vi "FGV Komponentenreferenzen verwalten.vi"(0 "Referenzen":refnum<vi>[](array[refnum]), 7 "Strings []":string[](array[string]), 11 "error in (no error)":errorcluster caption="Fehler (Eingang, kein Fehler)", 13 "Aktion":T1) -> (15 "error out":errorcluster caption="Fehler (Ausgang)")   [LabVIEW 2020, in "Linearisierung v2.lvlib" / "SpanEinstellungen.lvlib"]
uses:
  SpanEinstellungen.lvlib
  Aktion FGV Komponentenreferenz verwalten.ctl
  Gasteiler/HovaCAL_Interface/Kommunikation/Aktion FGV HovaCAL Interface Autolin.ctl
  Gasteiler/HovaCAL_Interface/Kommunikation/Kommunikation.lvlib
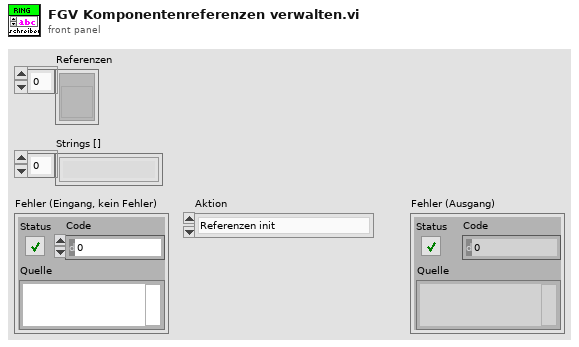
[diagram p1: front panel]
types:
  T1 = typedef "Linearisierung v2.lvlib/SpanEinstellungen.lvlib/Aktion FGV Komponentenreferenz verwalten.ctl" = enum16{"Referenzen init", "lesen", "Referenzen schließen", "Ring beschreiben", "MFC fix Werte setzen"}
  T2 = typedef "Linearisierung v2.lvlib/Gasteiler.lvlib/HovaCAL_Interface.lvlib/Kommunikation.lvlib/Aktion FGV HovaCAL Interface Autolin.ctl" = enum16{"lesen", "schreiben", "MFC Komponente fix setzen", "init"}
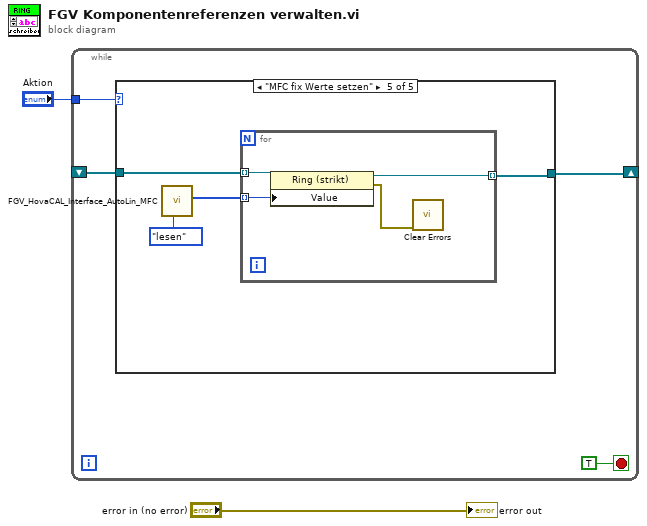
[diagram p0: block diagram]
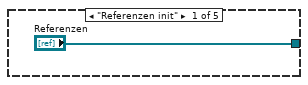
[diagram p2: hidden frame]
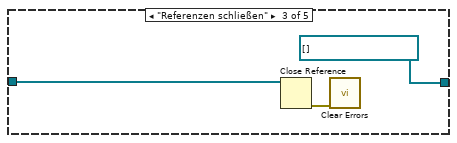
[diagram p4: hidden frame]
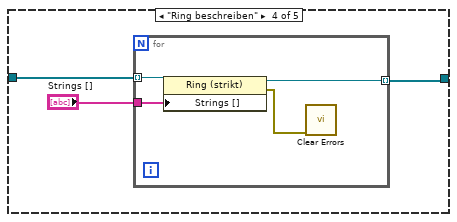
[diagram p5: hidden frame]
diagram:
  n1 = while {
    tunnel: "Aktion" -> [w6]
    shift-right: [w4] -> _
    shift-left: _ -> [w3]
    stop <- TRUE stop-if-true
    n2 = case shown="\"MFC fix Werte setzen\"" w6 {
      tunnel: ["Referenzen" w8 refnum<vi>[] [] ("Referenzen") w13 w21] -> w4
      tunnel: w3 -> [_ w8 w11 w14 w22]
      frame "Referenzen init" {
      }
      frame "lesen", Default {
      }
      frame "Referenzen schließen" {
        n3 = Close Reference(reference=w11) -> (error out=w9:errorcluster)  [unwired: 1 in]
        n4 = call <vilib>:"Clear Errors.vi"("error in (no error)"=w9) -> ()  [unwired: 5 in, 2 out]
      }
      frame "Ring beschreiben" {
        n5 = for {
          tunnel: w14 -> [w18] mode=indexing
          tunnel: [w17] -> w13 mode=indexing
          tunnel: "Strings []" -> [w15]
          n6 = property on="Eigenschaftsknoten" class="Ring (strikt)"(reference=w18, "Strings []"=w15) -> (reference out=w17:refnum<vi>, error out=w16:errorcluster)  [unwired: 1 in]
          n7 = call <vilib>:"Clear Errors.vi"("error in (no error)"=w16) -> ()  [unwired: 5 in, 2 out]
        }
      }
      frame "MFC fix Werte setzen" {
        n8 = call "FGV_HovaCAL_Interface_AutoLin_MFC.vi"("Aktion"=Aktion_FGV_HovaCAL_Interface_Autolin."lesen") -> ("MFV Komponente fix out"=w19:u16[])  [unwired: 7 in, 3 out]
        n9 = for {
          tunnel: w22 -> [w26] mode=indexing
          tunnel: [w25] -> w21 mode=indexing
          tunnel: w19 -> [w23] mode=indexing
          n10 = property on="Eigenschaftsknoten" class="Ring (strikt)"(reference=w26, "Value"=w23) -> (reference out=w25:refnum<vi>, error out=w24:errorcluster)  [unwired: 1 in]
          n11 = call <vilib>:"Clear Errors.vi"("error in (no error)"=w24) -> ()  [unwired: 5 in, 2 out]
        }
      }
    }
  }
  "error out" <- "error in (no error)"
